vi "Connect.vi"(8 "error in (no error)":errorcluster, 10 "conninfo":string) -> (0 "error out":errorcluster, 2 "PGconn":T1, 3 "PQ Connection out":refnum<class "PQ Connection.lvclass">)   [LabVIEW 2015, in "PQ Connection.lvclass"]
uses:
  PQ Connection.lvclass
  <vilib>/LAVA/libpq/Types/PGconn.ctl
  PQ Connection.lvclass/PQ Connection.ctl
  Error.vi
  <vilib>/LAVA/libpq/__lava_libpq.lvlib
  libpq.dll
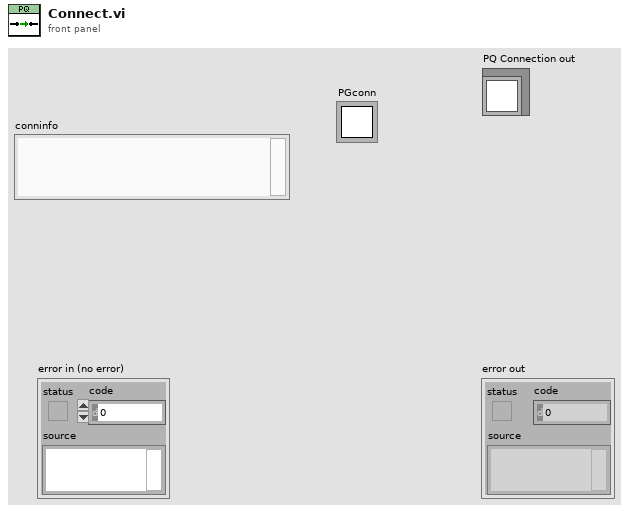
[diagram p1: front panel]
types:
  T1 = typedef "__lava_libpq.lvlib/PGconn.ctl" = refnum<k1>
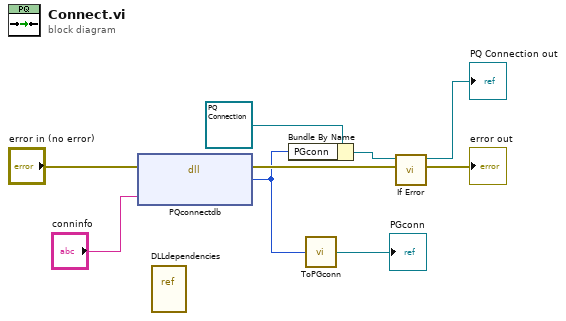
[diagram p0: block diagram]
diagram:
  n1 = dll-call lib="C:/PQ/Connection/libpq.dll" fn="PQconnectdb"(error in="error in (no error)", "conninfo"="conninfo") -> (error out=w6:errorcluster, "PGconn"=w1:u32)  [unwired: 3 in, 1 out]
  n2 = vi-ref <vilib>:"DLLdependencies.vi"() -> ()  [unwired: 1 out]
  n3 = Bundle By Name(cluster=refnum<class "PQ Connection.lvclass"> refnum ("PQ Connection in"), "PGconn"=w1) -> (w2:refnum<class "PQ Connection.lvclass">)
  n4 = call <vilib>:"ToPGconn.vi"("PGconn_ptr"=w1) -> ("PGconn"=→"PGconn":T1)
  n5 = call "If Error.vi"("error in (no error)"=w6, "PQ Connection in"=w2) -> ("error out"=→"error out":errorcluster, "PQ Connection out"=→"PQ Connection out":refnum<class "PQ Connection.lvclass">)  [unwired: 8 in]
